vi "Write Project Path.vi"(8 "error in (no error)":errorcluster, 10 "Project Path":path, 11 "LabVIEW Build Script in":refnum<class "LabVIEW Build Script.lvclass">) -> (0 "error out":errorcluster, 3 "LabVIEW Build Script out":refnum<class "LabVIEW Build Script.lvclass">)   [LabVIEW 2021, in "LabVIEW Build Script.lvclass"]
uses:
  LabVIEW Build Script.lvclass
  LabVIEW Build Script.lvclass/LabVIEW Build Script.ctl
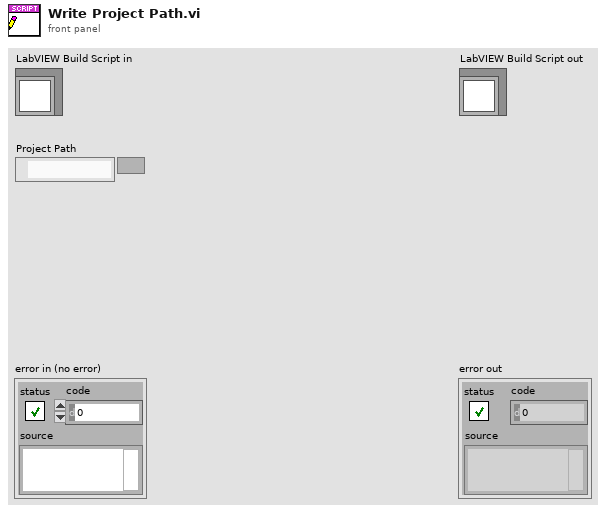
[diagram p1: front panel]
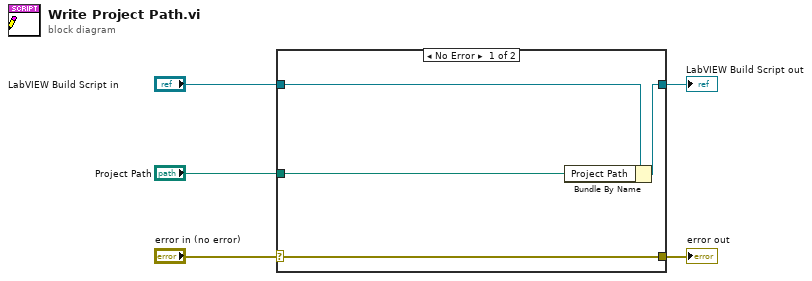
[diagram p0: block diagram]
diagram:
  n1 = case shown="No Error" "error in (no error)" {
    selector: "error in (no error)" -> [w9 w10]
    tunnel: [w9 w10] -> w4
    tunnel: [w7 w11] -> w2
    tunnel: "LabVIEW Build Script in" -> [w8 w11]
    tunnel: "Project Path" -> [w6 _]
    frame No Error {
      n2 = Bundle By Name(cluster=w8, "Project Path"=w6) -> (w7:refnum<class "LabVIEW Build Script.lvclass">)
    }
    frame Error {
    }
  }
  "error out" <- w4
  "LabVIEW Build Script out" <- w2
